vi "DataStream_RTQ_Write Q Data to Stream.vi"(8 "Error":errorcluster, 9 "Connected":bool, 10 "Time":i32=1000, 11 "Stream Writer Ref":T1) -> (0 "Error Out":errorcluster, 2 "Timed Out? Out":bool, 3 "Stream Writer Ref Out":T1)   [LabVIEW 2020]
uses:
  TypeDefs/Cluster_DataStream_RT Writer Refs.ctl
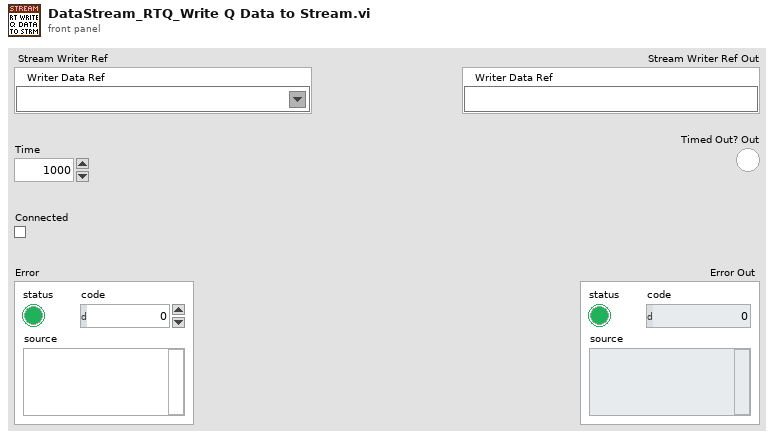
[diagram p1: front panel]
types:
  T1 = typedef "Cluster_DataStream_RT Writer Refs.ctl" = cluster{"Writer Data Ref":refnum<k21>}
  T2 = typedef "Cluster_DataStream RT Data Set.ctl" = cluster{"Header Array":string[], "Time Stamp Array":dbl[], "Value Array":dbl[]}
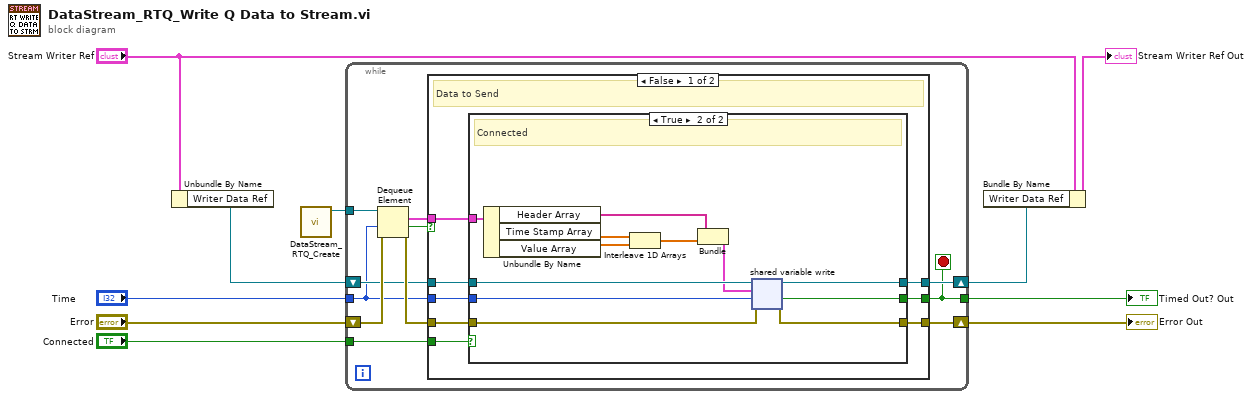
[diagram p0: block diagram]
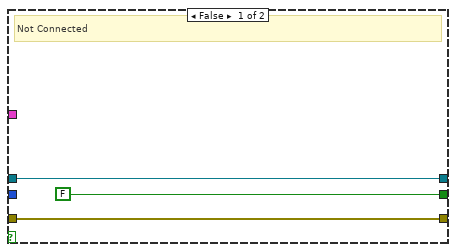
[diagram p2: hidden frame]
diagram:
  n1 = Unbundle By Name("Stream Writer Ref") -> ("Writer Data Ref"=w5:refnum<k21>)
  n2 = call "DataStream_RTQ_Create.vi"() -> ("RTQ"=w2:refnum<queue>)  [unwired: 11 in]
  n3 = while {
    tunnel: [w13] -> w4
    tunnel: "Time" -> [w14]
    shift-right: [w17] -> w8
    shift-left: "Error" -> [w16]
    shift-right: [w21] -> w9
    shift-left: w5 -> [w15]
    tunnel: w2 -> [w12]
    tunnel: "Connected" -> [w11]
    stop <- w13 stop-if-true
    n4 = Dequeue Element(queue=w12, timeout in ms (-1)=w14, error in (no error)=w16) -> (element=w18:T2, timed out?=w20:bool, error out=w19:errorcluster)  [unwired: 1 out]
    n5 = case shown="False" w20 {
      selector: w20 -> [_ w45]
      tunnel: [w29 w47] -> w21
      tunnel: w15 -> [w28 w47]
      tunnel: [w24 w46] -> w17
      tunnel: w18 -> [w26 _]
      tunnel: w19 -> [w27 w46]
      tunnel: [w25 w45] -> w13
      tunnel: w14 -> [w23 _]
      tunnel: w11 -> [w22 _]
      frame False {
        # "Data to Send"
        n6 = case shown="True" w22 {
          tunnel: [w32 w44] -> w29
          tunnel: w28 -> [w32 w43]
          tunnel: w27 -> [w30 w42]
          tunnel: w26 -> [_ w41]
          tunnel: [FALSE w40] -> w25
          tunnel: [w30 w38] -> w24
          tunnel: w23 -> [_ w39]
          frame False {
            # "Not Connected"
          }
          frame True {
            # "Connected"
            n7 = Unbundle By Name(w41) -> ("Header Array"=w37:string[], "Time Stamp Array"=w35:dbl[], "Value Array"=w34:dbl[])
            n8 = Interleave 1D Arrays(w35, w34) -> (w33:dbl[])
            n9 = Bundle("Header Array"=w37, w33) -> (w36:cluster{"Header Array":string[], dbl[]})  [unwired: 1 in]
            n10 = shared-variable-write(w43, w42, w36, w39) -> (w44:refnum<k21>, w38:errorcluster, w40:bool)
          }
        }
      }
      frame True {
        # "Timed Out No Data"
      }
    }
  }
  "Error Out" <- w8
  "Timed Out? Out" <- w4
  n11 = Bundle By Name(cluster="Stream Writer Ref", "Writer Data Ref"=w9) -> (→"Stream Writer Ref Out":T1)
